vi "Set Status Code.vi"(8 "error in (no error)":errorcluster, 10 "StatusCode":u16, 11 "net-response in":refnum<class "response.lvclass">) -> (0 "error out":errorcluster, 3 "net-response out":refnum<class "response.lvclass">)   [LabVIEW 2020, in "net-response.lvclass"]
uses:
  net-response.lvclass
  net-response.lvclass/net-response.ctl
  C:/Viviota/Projects/R&D/LabVIEW_HTTP_REST_Client/source/classes/response/response.lvclass
  C:/Viviota/Projects/R&D/LabVIEW_HTTP_REST_Client/source/net-response/net-response.lvclass
  classes/response/response.lvclass
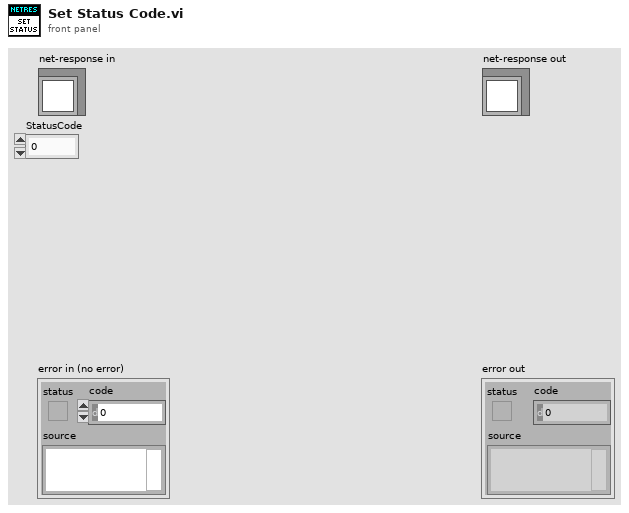
[diagram p1: front panel]
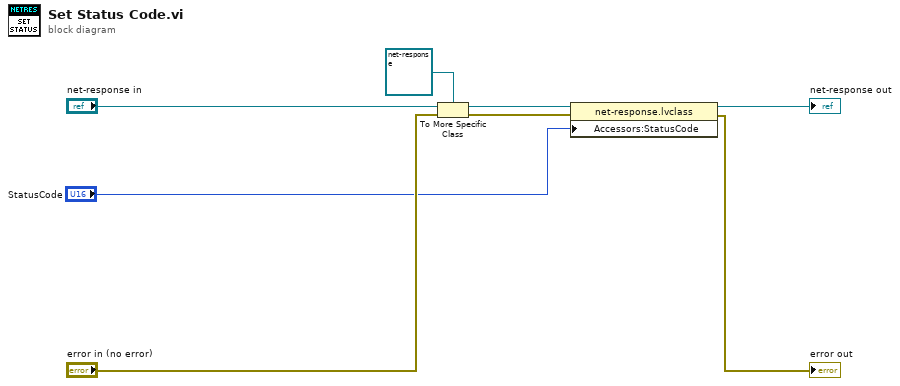
[diagram p0: block diagram]
diagram:
  n1 = To More Specific Class(target class=refnum<class "net-response.lvclass"> refnum ("net-response.lvclass"), reference="net-response in", error in="error in (no error)") -> (specific class reference=w7:refnum<class "net-response.lvclass">, error out=w2:errorcluster)
  n2 = property class="net-response.lvclass"(reference=w7, error in=w2, "Accessors:StatusCode"="StatusCode") -> (reference out=→"net-response out":refnum<class "net-response.lvclass">, error out=→"error out":errorcluster)
